vi "mSecToSec.vi"(11 "mSec":u32) -> (3 "Sec":dbl)   [LabVIEW 2013, in "Photometrics_CH-250_Cam.lvclass"]
uses:
  Photometrics_CH-250_Cam.lvclass
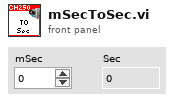
[diagram p1: front panel]
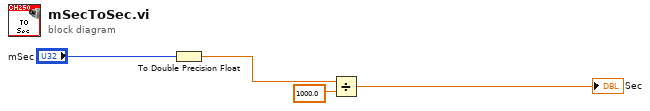
[diagram p0: block diagram]
diagram:
  n1 = To Double Precision Float(number="mSec") -> (double precision float=w1:dbl)
  n2 = Divide(x=w1, y=1000.0) -> (x/y=→"Sec":dbl)
